vi "choose-detection-exp.vi"() -> (0 "Type of experiment out":enum32{"Pump-probe", "Pump-push-probe"}(radio), 1 "Type of detection out":enum32{"IR detection", "UV-vis detection"}(radio))   [LabVIEW 2015]
panel:
  in  "Type of detection":enum32{"IR detection", "UV-vis detection"}(radio)
  in  "stop":bool
  in  "Type of experiment":enum32{"Pump-probe", "Pump-push-probe"}(radio)
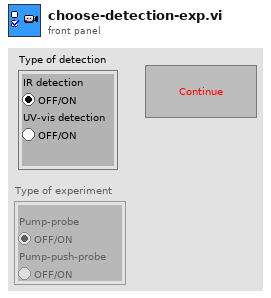
[diagram p1: front panel]
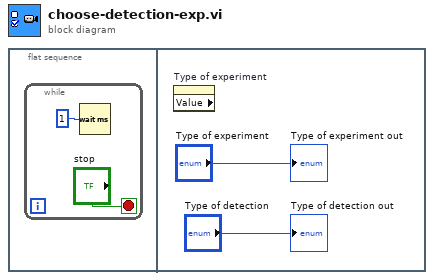
[diagram p0: block diagram]
diagram:
  n1 = flat-sequence {
    frame #0 {
      n2 = while {
        stop <- "stop" stop-if-true
        n3 = Wait (ms)(milliseconds to wait=u32 1) -> ()  [unwired: 1 out]
      }
    }
    frame #1 {
      n4 = property on="Type of experiment" class="CmdeBtnsRadio (strict)" props=["Value"]() -> ()  [unwired: 2 in, 3 out]
      "Type of detection out" <- "Type of detection"
      "Type of experiment out" <- "Type of experiment"
    }
  }
